vi "test_GetItemInfosFromProjectFile_SampleProject.vi"() -> (3 "Pass?":bool)   [LabVIEW 2019, in "Tests.SolutionBuilder.lvlib"]
uses:
  Tests.SolutionBuilder.lvlib
  SolutionBuilder/SolutionBuilder.lvclass
  SolutionBuilder/ProjectItem/ProjectItem.lvclass
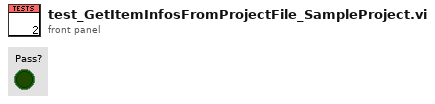
[diagram p1: front panel]
types:
  T1 = typedef "SolutionBuilder.lvlib/SolutionBuilder.lvclass/ProjectItemMap.ctl" = map{path, refnum<class "ProjectItem.lvclass">[]}
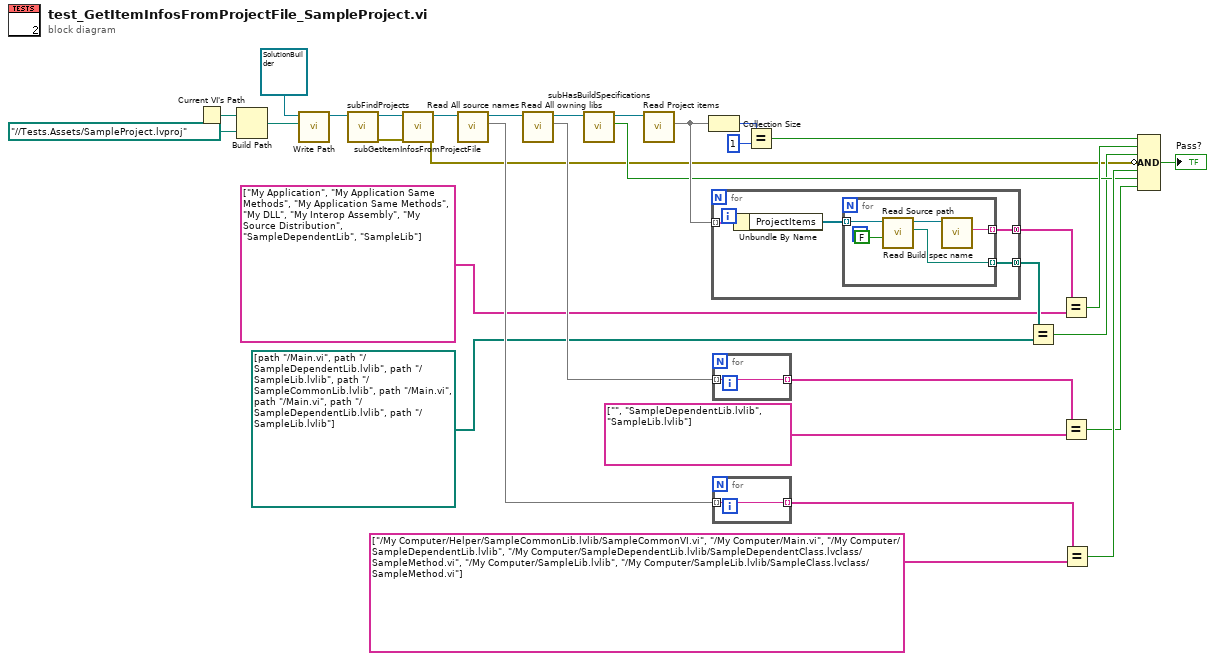
[diagram p0: block diagram]
diagram:
  n1 = Current VI's Path() -> (path=w29:path)
  n2 = Build Path(base path=w29, name or relative path=path "../../Tests.Assets/SampleProject.lvproj" ("Path")) -> (appended path=w27:path)
  n3 = call "Write Path.vi"("Path"=w27, "SolutionBuilder in"=refnum<class "SolutionBuilder.lvclass"> refnum) -> ("SolutionBuilder out"=w31:refnum<class "SolutionBuilder.lvclass">)  [unwired: 9 in]
  n4 = call "subFindProjects.vi"("SolutionBuilder in"=w31) -> ("error out"=w3:errorcluster, "SolutionBuilder out"=w30:refnum<class "SolutionBuilder.lvclass">)  [unwired: 9 in]
  n5 = call "subGetItemInfosFromProjectFile.vi"("error in (no error)"=w3, "SolutionBuilder in"=w30) -> ("error out"=w2:errorcluster, "SolutionBuilder out"=w24:refnum<class "SolutionBuilder.lvclass">)  [unwired: 8 in]
  n6 = call "Read All source names.vi"("SolutionBuilder in"=w24) -> ("All source names"=w20:set{string}, "SolutionBuilder out"=w11:refnum<class "SolutionBuilder.lvclass">)  [unwired: 9 in]
  n7 = call "Read All owning libs.vi"("SolutionBuilder in"=w11) -> ("All owning libs"=w9:set{string}, "SolutionBuilder out"=w10:refnum<class "SolutionBuilder.lvclass">)  [unwired: 9 in]
  n8 = call "subHasBuildSpecifications.vi"("SolutionBuilder in"=w10) -> ("Has specs?"=w17:bool, "SolutionBuilder out"=w18:refnum<class "SolutionBuilder.lvclass">)  [unwired: 8 in, 1 out]
  n9 = call "Read Project items.vi"("SolutionBuilder in"=w18) -> ("Project items"=w23:T1)  [unwired: 9 in, 1 out]
  n10 = Collection Size(1:w23) -> (0:w26:i32)
  n11 = for {
    tunnel: w23 -> [w36] mode=indexing
    tunnel: [w35] -> w16 mode=concatenating
    tunnel: [w33] -> w13 mode=concatenating
    n12 = Unbundle By Name(w36) -> ("ProjectItems"=w34:refnum<class "ProjectItem.lvclass">[])
    n13 = for {
      tunnel: w34 -> [w39] mode=indexing
      tunnel: [w41] -> w35 mode=indexing
      tunnel: [w38] -> w33 mode=indexing
      n14 = call "Read Source path.vi"("Force abs path? (T)"=FALSE, "ProjectItem in"=w39) -> ("Source path"=w38:path, "ProjectItem out"=w40:refnum<class "ProjectItem.lvclass">)  [unwired: 8 in]
      n15 = call "Read Build spec name.vi"("ProjectItem in"=w40) -> ("Build spec name"=w41:string)  [unwired: 9 in, 1 out]
    }
  }
  n16 = for {
    tunnel: w9 -> [w42] mode=indexing
    tunnel: [w42] -> w8 mode=indexing
  }
  n17 = for {
    tunnel: w20 -> [w43] mode=indexing
    tunnel: [w43] -> w15 mode=indexing
  }
  n18 = Equal?(x=w26, y=1) -> (x = y?=w22:bool)
  n19 = Equal?(x=w13, y=path[] [path "../Main.vi", path "../SampleDependentLib.lvlib", path "../SampleLib.lvlib", path "../SampleCommonLib.lvlib", path "../Main.vi", path "../Main.vi", path "../SampleDependentLib.lvlib", path "../SampleLib.lvlib"] ("Array 2")) -> (x = y?=w12:bool)
  n20 = Equal?(x=w16, y=string[] ["My Application", "My Application Same Methods", "My Application Same Methods", "My DLL", "My Interop Assembly", "My Source Distribution", "SampleDependentLib", "SampleLib"] ("Array")) -> (x = y?=w21:bool)
  n21 = Equal?(x=w8, y=string[] ["", "SampleDependentLib.lvlib", "SampleLib.lvlib"] ("Array")) -> (x = y?=w6:bool)
  n22 = Equal?(x=w15, y=string[] ["/My Computer/Helper/SampleCommonLib.lvlib/SampleCommonVI.vi", "/My Computer/Main.vi", "/My Computer/SampleDependentLib.lvlib", "/My Computer/SampleDependentLib.lvlib/SampleDependentClass.lvclass/SampleMethod.vi", "/My Computer/SampleLib.lvlib", "/My Computer/SampleLib.lvlib/SampleClass.lvclass/SampleMethod.vi"] ("Array 2")) -> (x = y?=w19:bool)
  n23 = Compound Arithmetic op=AND(w22, w21, w12, invert w2, w19, w17, w6) -> (→"Pass?":bool)
